vi "n_edge.vi"(11 "in":bool) -> (3 "out":bool)   [LabVIEW 2012]
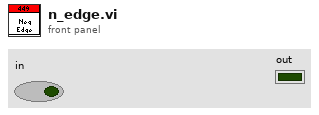
[diagram p1: front panel]
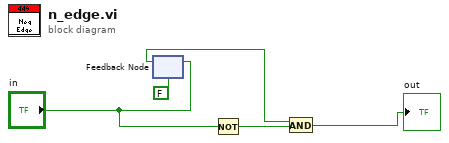
[diagram p0: block diagram]
diagram:
  n1 = feedback-in #1("in") -> ()
  n2 = feedback #1(FALSE ("in")) -> (w1:bool)
  n3 = Not(x="in") -> (.not. x?=w3:bool)
  n4 = And(x=w1, y=w3) -> (x .and. y?=→"out":bool)
